vi "Get Temp Directory.vi"(7 "Flush Files (F)":bool, 8 "error in (no error)":errorcluster, 11 "Dir path":path) -> (0 "error out":errorcluster, 2 "Exists?":bool, 3 "created path":path)   [LabVIEW 2019, in "Exaprom PDF.lvlib"]
doc: "If Dir path is empty then we utilize the default directory (for Vista: users\\%USERPROFILE%\\AppData\\Local\\Temp)\n\nVersion 1.0\nDeveloped by Jean-Marc Simard\nCopyright © 2010, Exaprom Inc.\nAll rights reserved.\nLicense: BSD"
uses:
  Exaprom PDF.lvlib
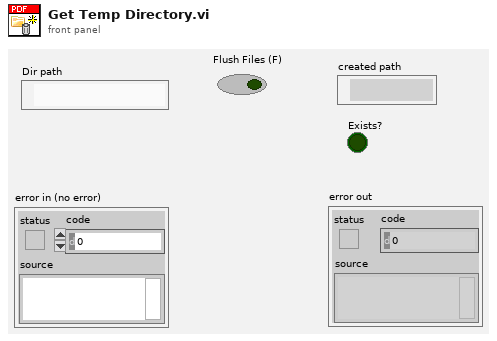
[diagram p1: front panel]
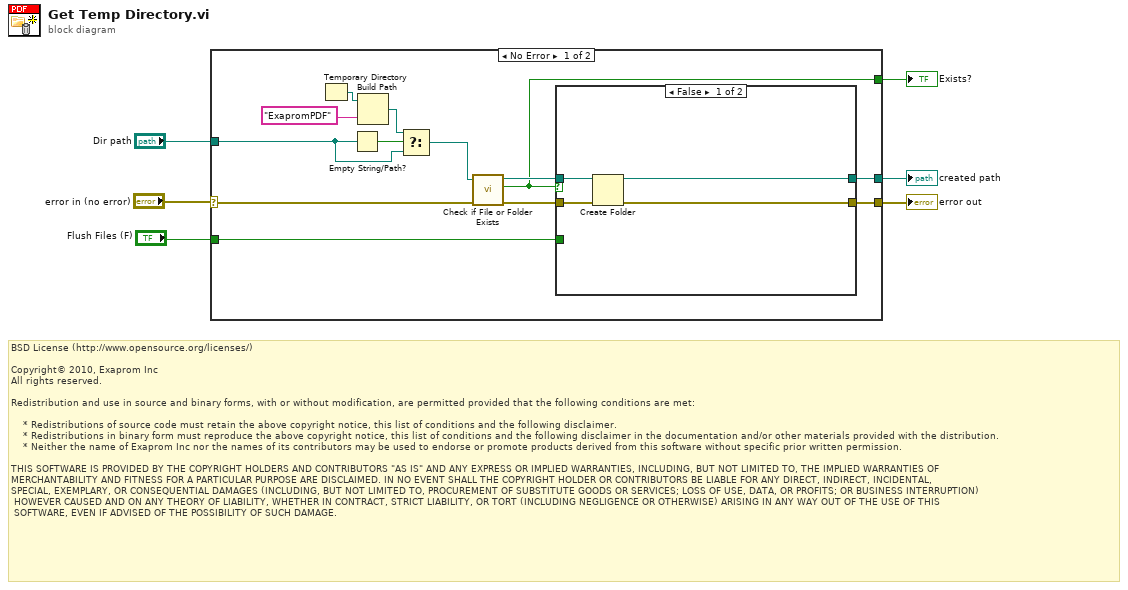
[diagram p0: block diagram]
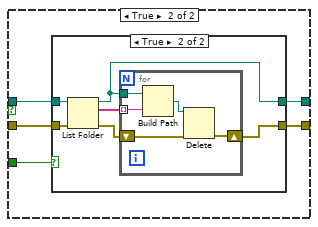
[diagram p2: hidden frame]
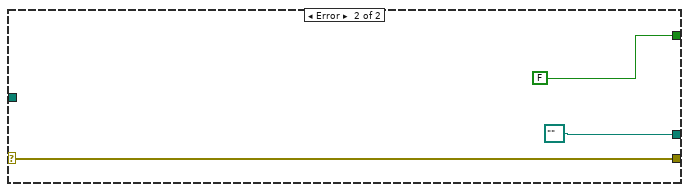
[diagram p4: hidden frame]
diagram:
  # "BSD License (http://www.opensource.org/licenses/)\n\nCopyright© 2010, Exaprom Inc\nAll rights reserved.\n\nRedistribution and use in source and binary forms, with or without modification, are permitted provided that the following conditions are met:\n\n    * Redistributions of source code must retain the above copyright notice, this list of conditions and the following disclaimer.\n    * Redistributions in binary form must reproduce the above copyright notice, this list of conditions and the following disclaimer in the documentation and/or other materials provided with the distribution.\n    * Neither the name of Exaprom Inc nor the names of its contributors may be used to endorse or promote products derived from this software without specific prior written permission.\n\nTHIS SOFTWARE IS PROVIDED BY THE COPYRIGHT HOLDERS AND CONTRIBUTORS \"AS IS\" AND ANY EXPRESS OR IMPLIED WARRANTIES, INCLUDING, BUT NOT LIMITED TO, THE IMPLIED WARRANTIES OF \nMERCHANTABILITY AND FITNESS FOR A PARTICULAR PURPOSE ARE DISCLAIMED. IN NO EVENT SHALL THE COPYRIGHT HOLDER OR CONTRIBUTORS BE LIABLE FOR ANY DIRECT, INDIRECT, INCIDENTAL,\nSPECIAL, EXEMPLARY, OR CONSEQUENTIAL DAMAGES (INCLUDING, BUT NOT LIMITED TO, PROCUREMENT OF SUBSTITUTE GOODS OR SERVICES; LOSS OF USE, DATA, OR PROFITS; OR BUSINESS INTERRUPTION)\n HOWEVER CAUSED AND ON ANY THEORY OF LIABILITY, WHETHER IN CONTRACT, STRICT LIABILITY, OR TORT (INCLUDING NEGLIGENCE OR OTHERWISE) ARISING IN ANY WAY OUT OF THE USE OF THIS\n SOFTWARE, EVEN IF ADVISED OF THE POSSIBILITY OF SUCH DAMAGE."
  n1 = case shown="No Error" "error in (no error)" {
    selector: "error in (no error)" -> [w17 w44]
    tunnel: [w16 w44] -> w6
    tunnel: [w15 path "" ("dup path")] -> w4
    tunnel: [w14 FALSE ("file or folder exists?")] -> w3
    tunnel: "Flush Files (F)" -> [w13 _]
    tunnel: "Dir path" -> [w11 _]
    frame No Error {
      n2 = Temporary Directory() -> (w10:path)
      n3 = Empty String/Path?(string/path=w11) -> (empty?=w12:bool)
      n4 = Build Path(base path=w10, name or relative path="ExapromPDF") -> (appended path=w9:path)
      n5 = Select(t=w9, s=w12, f=w11) -> (s? t:f=w7:path)
      n6 = call <vilib>:"Check if File or Folder Exists.vi"("error in (no error)"=w17, "path"=w7) -> ("error out"=w18:errorcluster, "file or folder exists?"=w14:bool, "dup path"=w19:path)  [unwired: 7 out]
      n7 = case shown="False" w14 {
        tunnel: w19 -> [w23 w27]
        tunnel: w18 -> [w22 w28]
        tunnel: [w21 w25] -> w16
        tunnel: [w20 w26] -> w15
        tunnel: w13 -> [_ w24]
        frame False {
          n8 = Create Folder(path (use dialog)=w23, error in=w22) -> (created path=w20:path, error out=w21:errorcluster)  [unwired: 2 out]
        }
        frame True {
          n9 = case shown="True" w24 {
            tunnel: w28 -> [w29 w36]
            tunnel: w27 -> [w30 w35]
            tunnel: [w30 w33] -> w26
            tunnel: [w29 w31] -> w25
            frame False {
            }
            frame True {
              n10 = List Folder(path=w35, error in=w36) -> (path out=w33:path, filenames=w34:string[], error out=w32:errorcluster)  [unwired: 3 out]
              n11 = for {
                shift-right: [w40] -> w31
                shift-left: w32 -> [w41]
                tunnel: w34 -> [w39] mode=indexing
                tunnel: w33 -> [w38]
                n12 = Build Path(base path=w38, name or relative path=w39) -> (appended path=w37:path)
                n13 = Delete(path (use dialog)=w37, error in=w41) -> (error out=w40:errorcluster)  [unwired: 5 out]
              }
            }
          }
        }
      }
    }
    frame Error {
    }
  }
  "error out" <- w6
  "created path" <- w4
  "Exists?" <- w3
